vi "TestNewmarkOpenCloseNET.vi"() -> ()   [LabVIEW 2020]
panel:
  out "error out 2":errorcluster
  in  "error in (no error)":errorcluster
  out "error out":errorcluster
  out "connection":string
  out "libraryVersion":string
  in  "address":string="192.168.17.226"
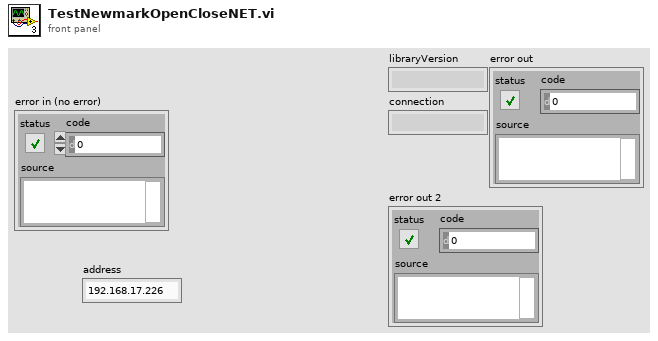
[diagram p1: front panel]
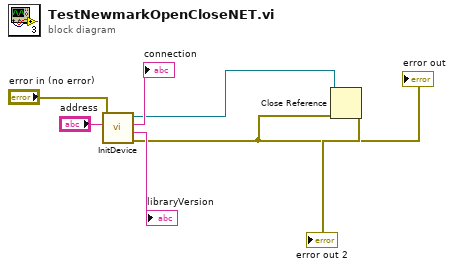
[diagram p0: block diagram]
diagram:
  n1 = call "InitDevice.vi"("error in (no error)"="error in (no error)", "address"="address") -> ("error out"=w1:errorcluster, "libraryVersion"=→"libraryVersion":string, "connection"=→"connection":string, "reference out"=w3:refnum<k7>)  [unwired: 6 in]
  "error out" <- w1
  n2 = Close Reference(reference=w3, error in (no error)=w1) -> (error out=→"error out 2":errorcluster)
